vi "生成校准信息.vi"(7 "table输入":string="总氮", 10 "量程下拉列表":refnum<vi>, 11 "曲线模型":refnum<vi>) -> ()   [LabVIEW 2016, in "斯坦道总氮.lvlib"]
panel:
  out "量程选择":enum16{"低量程", "高量程"}(ring)
  out "公式系数":cluster{"X^2":dbl, "K":dbl, "B":dbl, "R^2":dbl}
  out "校准时间":timestamp[](array[timestamp])
  out "启用":bool[](array[boolean])
  out "信号值":dbl[](array[numeric])
  out "校准浓度":dbl[](array[numeric])
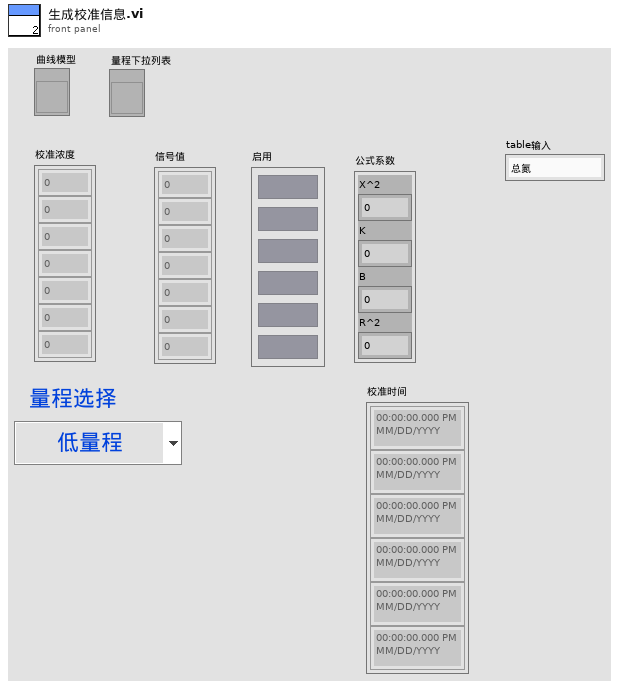
[diagram p1: front panel]
types:
  T1 = cluster{"时间标识":timestamp, "参数":string, "日志信息":string, "流程参数":string}
  T2 = cluster{"标液浓度1":dbl, "标液浓度2":dbl, "标液浓度3":dbl, "标液浓度4":dbl, "标液浓度5":dbl}
  T3 = cluster{"Value":dbl, "Value 2":dbl, "Value 3":dbl, "Value 4":dbl, "Value 5":dbl}
  T4 = cluster{"零点校准时间":timestamp, "标液校准时间1":timestamp, "标液校准时间2":timestamp, "标液校准时间3":timestamp, "标液校准时间4":timestamp}
  T5 = cluster{"启用":bool, "启用 2":bool, "启用 3":bool, "启用 4":bool, "启用 5":bool}
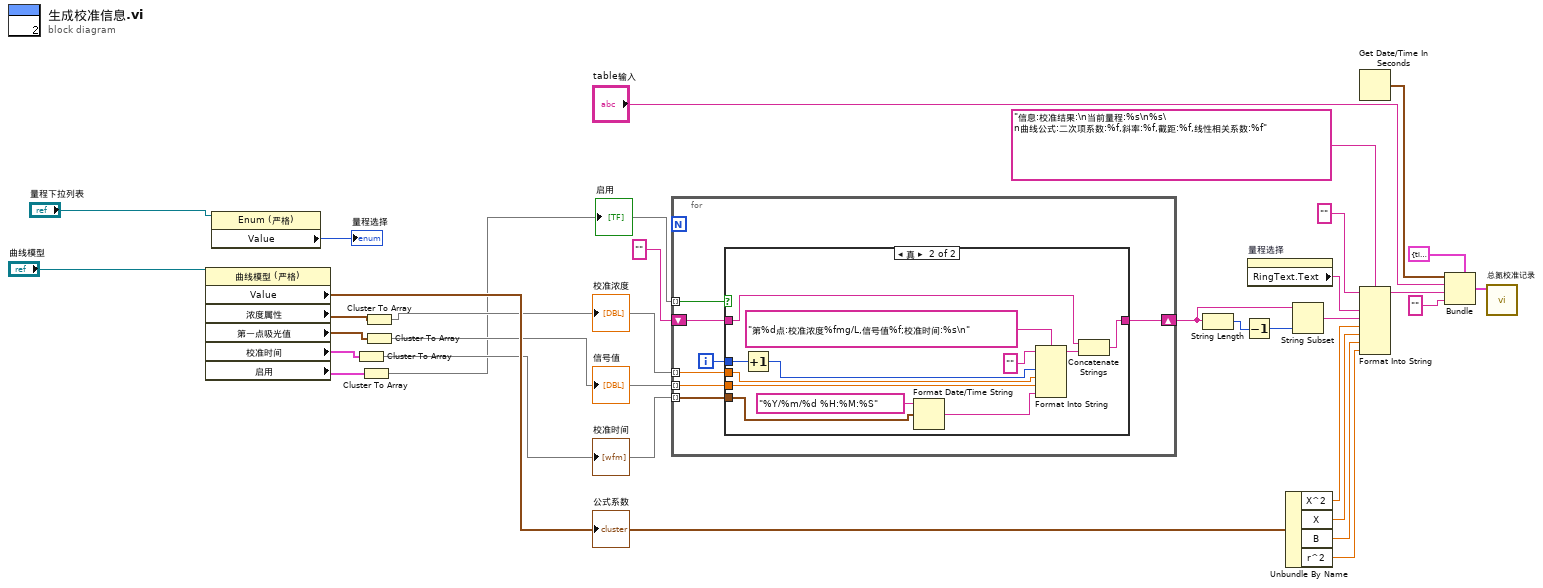
[diagram p0: block diagram]
diagram:
  n1 = property class="曲线模型 (严格)"(reference="曲线模型") -> ("Value"=w6:cluster{"X^2":dbl, "X":dbl, "B":dbl, "r^2":dbl}, "浓度属性"=w12:T2, "第一点吸光值"=w11:T3, "校准时间"=w10:T4, "启用"=w9:T5)  [unwired: 1 in, 2 out]
  "公式系数" <- w6
  n2 = property class="Enum (严格)"(reference="量程下拉列表") -> ("Value"=→"量程选择":enum16{"低量程", "高量程"})  [unwired: 1 in, 2 out]
  n3 = Cluster To Array(cluster=w10) -> (array=w2:timestamp[])
  "校准时间" <- w2
  n4 = Cluster To Array(cluster=w9) -> (array=w1:bool[])
  "启用" <- w1
  n5 = Cluster To Array(cluster=w12) -> (array=w4:dbl[])
  "校准浓度" <- w4
  n6 = Cluster To Array(cluster=w11) -> (array=w3:dbl[])
  "信号值" <- w3
  n7 = for {
    tunnel: w1 -> [w37] mode=indexing
    tunnel: w4 -> [w35] mode=indexing
    tunnel: w3 -> [w34] mode=indexing
    shift-right: [w33] -> w27
    shift-left: "" -> [w32]
    tunnel: w2 -> [w31] mode=indexing
    i -> [w36]
    n8 = case shown="真" w37 {
      tunnel: w36 -> [_ w48]
      tunnel: w35 -> [_ w47]
      tunnel: w34 -> [_ w46]
      tunnel: [w38 w43] -> w33
      tunnel: w32 -> [w38 w42]
      tunnel: w31 -> [_ w40]
      frame False {
      }
      frame True {
        n9 = Increment(x=w48) -> (x+1=w49:i32)
        n10 = Format Date/Time String(time format string (%c)="%Y/%m/%d %H:%M:%S" ("时间格式字符串(%c)"), seconds (now)=w40) -> (date/time string=w39:string)  [unwired: 1 in]
        n11 = Format Into String(format string="第%d点:校准浓度%fmg/L,信号值%f;校准时间:%s\n" ("格式字符串"), initial string="" ("初始字符串"), w49, w47, w46, w39) -> (resulting string=w44:string)  [unwired: 1 in, 1 out]
        n12 = Concatenate Strings(w42, w44) -> (w43:string)
      }
    }
  }
  n13 = String Length(string=w27) -> (length=w26:i32)
  n14 = Decrement(x=w26) -> (x-1=w25:i32)
  n15 = property on="量程选择" class="Enum (严格)"() -> ("RingText.Text"=w15:string)  [unwired: 2 in, 2 out]
  n16 = Unbundle By Name(w6) -> ("X^2"=w24:dbl, "X"=w23:dbl, "B"=w22:dbl, "r^2"=w13:dbl)
  n17 = String Subset(string=w27, length (rest)=w25) -> (substring=w16:string)  [unwired: 1 in]
  n18 = Get Date/Time In Seconds() -> (seconds since 1Jan1904=w19:timestamp)
  n19 = Format Into String(format string="信息:校准结果:\n当前量程:%s\n%s\n曲线公式:二次项系数:%f,斜率:%f,截距:%f,线性相关系数:%f", initial string="" ("初始字符串"), w15, w16, w24, w23, w22, w13) -> (resulting string=w17:string)  [unwired: 1 in, 1 out]
  n20 = Bundle(cluster=T1 {"时间标识"=timestamp(0 s since 1904-01-01), "参数"="", "日志信息"="", "流程参数"=""} ("data in"), "时间标识"=w19, "参数"="table输入", "日志信息"=w17, "流程参数"="" ("table输入")) -> (w14:T1)
  n21 = call "总氮校准记录.vi"("data in"=w14) -> ()  [unwired: 11 in]
